vi "Get Transfer Groups.vi"(11 "Cache in":refnum<class "Memory Cache.lvclass">) -> (2 "Transfers Groups":refnum<class "DSF.Engine.Transfer Group.lvclass">[](array[class]), 3 "Cache out":refnum<class "Memory Cache.lvclass">)   [LabVIEW 2017, in "Data Sharing Framework Engine.lvlib" / "Memory Cache.lvclass"]
uses:
  Memory Cache.lvclass
  old/dsf core/Source/Engine/Classes/Transfer/DSF.Engine.Transfer Group.lvclass
  Memory Cache.lvclass/Memory Cache.ctl
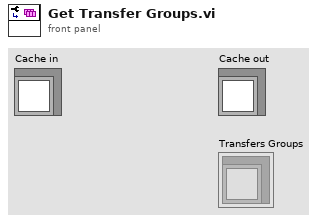
[diagram p1: front panel]
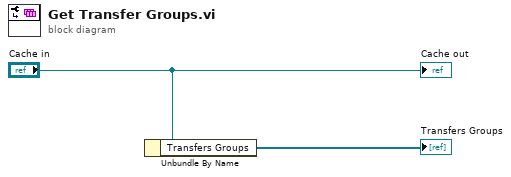
[diagram p0: block diagram]
diagram:
  n1 = Unbundle By Name("Cache in") -> ("Transfers Groups"=→"Transfers Groups":refnum<class "DSF.Engine.Transfer Group.lvclass">[])
  "Cache out" <- "Cache in"
